vi "MGI Get Handler Description.vi"(11 "MGI Error Handler in":refnum<class "MGI Error Reporter Dialog.lvclass">) -> (2 "Handler Description":string, 3 "MGI Error Handler out":refnum<class "MGI Error Reporter Dialog.lvclass">)   [LabVIEW 2016, in "MGI Error Reporter Dialog.lvclass"]
doc: "Output a string that describes the behavior of the error handler. This string is displayed in the Message string of the error handler window. This VI outputs a string the explains where the error directory is, how many errors are logged, and how many error logs are kept.\n\nAuthored by Shawn Walpole\nsupport@mooregoodideas.com\nwww.mooregoodideas.com\n\nCopyright (c) 2013, Moore Good Ideas, Inc.\n\nAll rights reserved.\n\nRedistribution and use in source and binary forms, with or without modification, are permitted provided that the following conditions are met:\n\n * Redistributions of source code must retain the above copyright notice, this list of conditions and the following disclaimer.\n * Redistributions in binary form must reproduce the above copyright notice, this list of conditions and the following disclaimer in the documentation and/or other materials provided with the distribution.\n * Neither the name of Moore Good Ideas, Inc. nor the names of its contributors may be used to endorse or promote products derived from this software without specific prior written permission.\n\nTHIS SOFTWARE IS PROVIDED BY THE COPYRIGHT HOLDERS AND CONTRIBUTORS \"AS IS\" AND ANY EXPRESS OR IMPLIED WARRANTIES, INCLUDING, BUT NOT LIMITED TO, THE IMPLIED WARRANTIES OF MERCHANTABILITY AND FITNESS FOR A PARTICULAR PURPOSE ARE DISCLAIMED. IN NO EVENT SHALL THE COPYRIGHT OWNER OR CONTRIBUTORS BE LIABLE FOR ANY DIRECT, INDIRECT, INCIDENTAL, SPECIAL, EXEMPLARY, OR CONSEQUENTIAL DAMAGES (INCLUDING, BUT NOT LIMITED TO, PROCUREMENT OF SUBSTITUTE GOODS OR SERVICES; LOSS OF USE, DATA, OR PROFITS; OR BUSINESS INTERRUPTION) HOWEVER CAUSED AND ON ANY THEORY OF LIABILITY, WHETHER IN CONTRACT, STRICT LIABILITY, OR TORT (INCLUDING NEGLIGENCE OR OTHERWISE) ARISING IN ANY WAY OUT OF THE USE OF THIS SOFTWARE, EVEN IF ADVISED OF THE POSSIBILITY OF SUCH DAMAGE."
uses:
  <userlib>/_MGI/Error Reporter/MGI Error Reporter Dialog/MGI Error Reporter Dialog.lvclass
  C:/Program Files (x86)/National Instruments/LabVIEW 2016/user.lib/_MGI/Error Reporter/MGI Error Reporter Base/MGI Error Reporter Base.lvclass
  <userlib>/_MGI/Error Reporter/MGI Error Reporter Base/MGI Error Reporter Base.lvclass
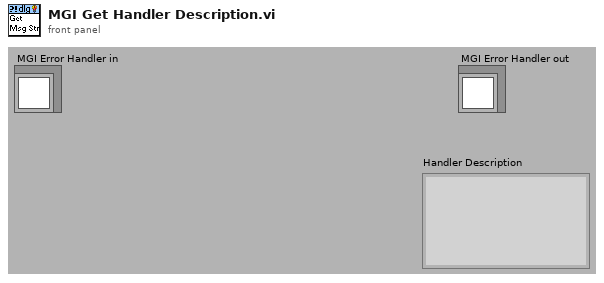
[diagram p1: front panel]
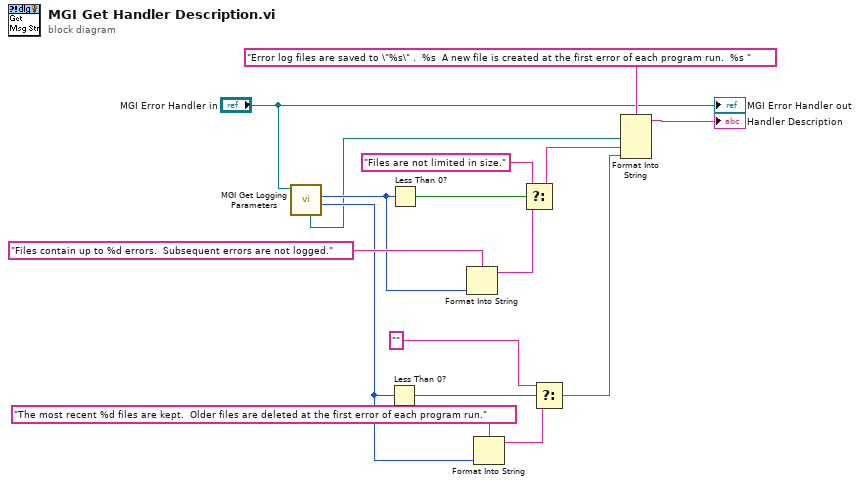
[diagram p0: block diagram]
diagram:
  n1 = call <userlib>:"MGI Get Logging Parameters.vi"("MGI Error Reporter Base"="MGI Error Handler in") -> ("Max # Log Files"=w2:i32, "Max # Errors to Log"=w3:i32, "Error Log Directory"=w1:path)  [unwired: 8 out]
  n2 = Less Than 0?(x=w2) -> (x < 0?=w14:bool)
  n3 = Less Than 0?(x=w3) -> (x < 0?=w15:bool)
  n4 = Format Into String(format string="Files contain up to %d errors.  Subsequent errors are not logged.", w3) -> (resulting string=w10:string)  [unwired: 2 in, 1 out]
  n5 = Format Into String(format string="The most recent %d files are kept.  Older files are deleted at the first error of each program run.", w2) -> (resulting string=w6:string)  [unwired: 2 in, 1 out]
  n6 = Select(t="Files are not limited in size.", s=w15, f=w10) -> (s? t:f=w11:string)
  n7 = Select(t="", s=w14, f=w6) -> (s? t:f=w9:string)
  n8 = Format Into String(format string="Error log files are saved to \"%s\" .  %s  A new file is created at the first error of each program run.  %s ", w1, w11, w9) -> (resulting string=→"Handler Description":string)  [unwired: 2 in, 1 out]
  "MGI Error Handler out" <- "MGI Error Handler in"
